vi "FringeTracker-AlignRaster.vi"(0 "error in (no error)":errorcluster, 2 "FringeTracker name":string="RTC21Summit.RTC.FringeTracker.0") -> (3 "error out":errorcluster, 7 "xOffset":dbl, 9 "yOffset":dbl)   [LabVIEW 2009]
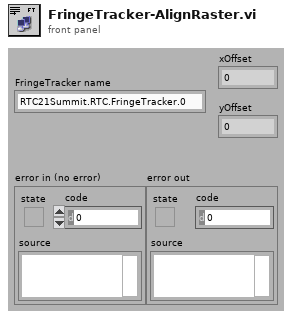
[diagram p1: front panel]
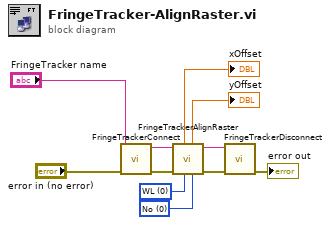
[diagram p0: block diagram]
diagram:
  w4 = 0 items=["No", "Yes"] ("goToPeak")
  w5 = 0 items=["WL", "SPEC"] ("channel")
  n1 = call "FringeTrackerConnect.vi"("FringeTracker Name"="FringeTracker name", "error in (no error)"="error in (no error)") -> ("FringeTracker Name out"=w8:string, "error out"=w11:errorcluster)  [unwired: 6 out]
  n2 = call "FringeTrackerAlignRaster.vi"("goToPeak"=w4, "channel"=w5, "error in (no error)"=w11, "FringeTracker Name"=w8) -> ("error out"=w10:errorcluster, "FringeTracker Name out"=w9:string, "yOffset"=→"yOffset":dbl, "xOffset"=→"xOffset":dbl)  [unwired: 4 out]
  n3 = call "FringeTrackerDisconnect.vi"("FringeTracker Name"=w9, "error in (no error)"=w10) -> ("error out"=→"error out":errorcluster)  [unwired: 7 out]
